vi "addSeparator.vi"(8 "Error In":errorcluster, 11 "QWinJumpListCategory In":refnum<class "QWinJumpListCategory.lvclass">) -> (0 "Error Out":errorcluster, 2 "Value":refnum<class "QWinJumpListItem.lvclass">, 3 "QWinJumpListCategory Out":refnum<class "QWinJumpListCategory.lvclass">)   [LabVIEW 2014, in "QWinJumpListCategory.lvclass"]
doc: "LabVIEW-specific documentation is not yet available."
uses:
  QWinJumpListCategory.lvclass
  QWinJumpListItem/QWinJumpListItem.lvclass
  LQ Core/LQIdentity/LQIdentity.lvclass/LQIdentity.ctl
  LQ Core/LQ Core.lvlib
  LQ Core/LQIdentity/LQIdentity.lvclass
  LQ Core/LQCoreEngine/LQCoreEngine.lvclass
panel:
  # "Copyright (c) 2016 Sze Howe Koh\n\nThis Source Code Form is subject to the terms of the Mozilla Public\nLicense, v. 2.0. If a copy of the MPL was not distributed with this\nfile, You can obtain one at http://mozilla.org/MPL/2.0/."
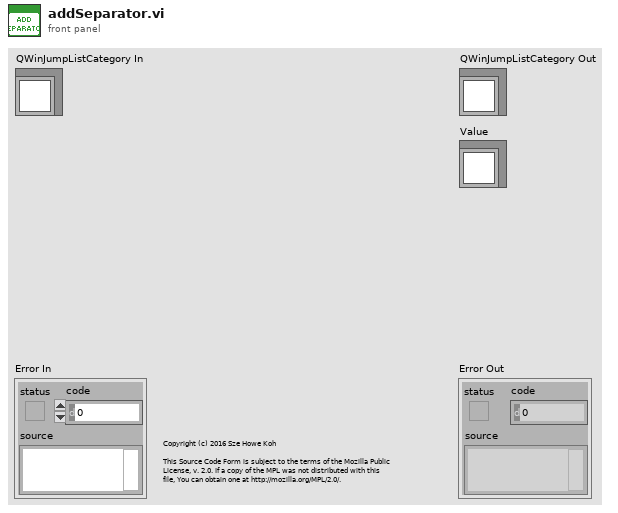
[diagram p1: front panel]
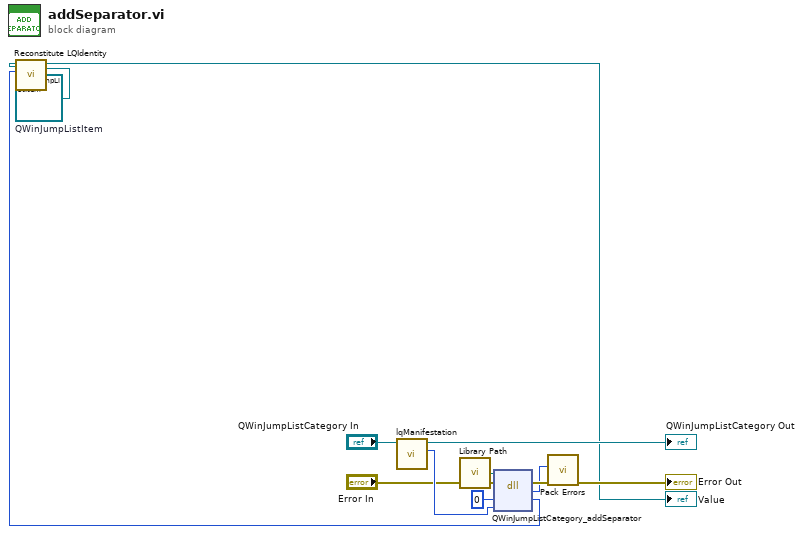
[diagram p0: block diagram]
diagram:
  w1 = refnum<class "QWinJumpListItem.lvclass"> refnum  # QWinJumpListItem
  n1 = call "lqManifestation.vi"("LQIdentity in"="QWinJumpListCategory In") -> ("Manifestation"=w8:u64, "LQIdentity out"=→"QWinJumpListCategory Out":refnum<class "QWinJumpListCategory.lvclass">)  [unwired: 9 in]
  n2 = call "Library Path.vi"() -> ("Library Path"=w9:path)
  n3 = dll-call lib="?" fn="QWinJumpListCategory_addSeparator"(path in=w9, error in="Error In", "_retVal"=u64 0 ("retVal"), "_instance"=w8) -> (error out=w6:errorcluster, w4:i32, "_retVal"=w2:u64)  [unwired: 2 in, 1 out]
  n4 = call "Reconstitute LQIdentity.vi"("Manifestation"=w2, "LQIdentity Prototype"=w1) -> ("Reconstituted LQIdentity"=→"Value":refnum<class "QWinJumpListItem.lvclass">)  [unwired: 8 in, 1 out]
  n5 = call "Pack Errors.vi"("Error In"=w6, "Error Code"=w4) -> ("Error Out"=→"Error Out":errorcluster)  [unwired: 9 in]
